vi "error handler - SubVI.vi"(4 "error in":errorcluster, 7 "Dialog box?":bool=TRUE) -> (0 "error out":errorcluster, 2 "message":string=" INSTRUCTIONS:\r\rNormal Use:  When using subVIs that incorporate the error in/error out (or error I/O) structure, place this handler where you want to inform the user of an error, typically at the end of the I/O data path, as the last action of the program.  If the error in error? is ERROR, the handler creates a message describing the error and its source.  If the type of dialog = 1 (default), the message is displayed to the user, who can only acknowedge it.  If the type = 2, the user can acknowledge the message or abort execution; aborting a program with active I/O is not recommended.  If the type = 0, no message is displayed; this is used to process the error programmatically, and the error out cluster elements are wired to individual terminals for that reason.  \r\rOther Use:\n\r\nlocal testing.  To test the error code of a subVI or function that does not have the error I/O structure, you can wire its error code and a source string to the local error code and error source inputs.  If error in error? indicates no error and error code is not equal to 0, the local code and source are substituted for the error in values, and error? is set TRUE (ERROR).", 3 "no error out":errorcluster)   [LabVIEW 2014]
uses:
  Lambda Globals.vi
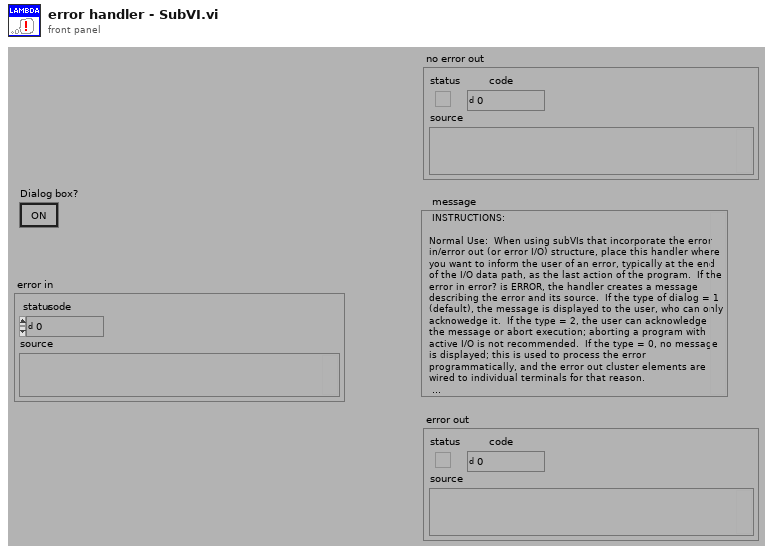
[diagram p1: front panel]
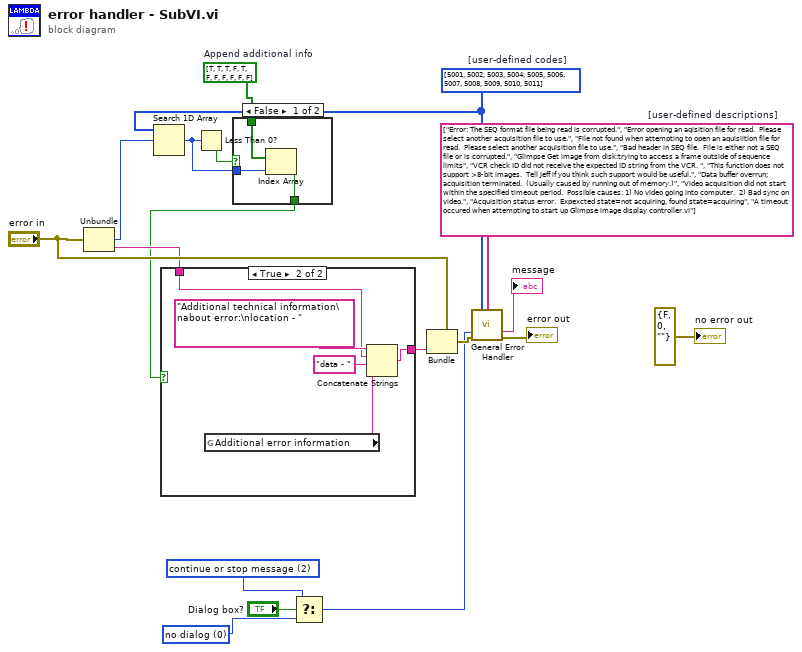
[diagram p0: block diagram]
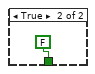
[diagram p2: hidden frame]
diagram:
  w5 = u16 2 items=["no dialog", "OK message", "continue or stop message"] ("type of dialog (OK msg:1)")
  w4 = u16 0 items=["no dialog", "OK message", "continue or stop message"] ("type of dialog (OK msg:1)")
  w8 = bool[] [TRUE, TRUE, TRUE, FALSE, TRUE, FALSE, FALSE, FALSE, FALSE, FALSE, FALSE]  # Append additional info
  w17 = string[] ["Error: The SEQ format file being read is corrupted.", "Error opening an aqisition file for read.  Please select another acquisition file to use.", "File not found when attempting to open an aquisiition file for read.  Please select another acquisition file to use.", "Bad header in SEQ file.  File is either not a SEQ file or is corrupted.", "Glimpse Get image from disk:trying to access a frame outside of sequence limits", "VCR check ID did not receive the expected ID string from the VCR. ", "This function does not support >8-bit images.  Tell Jeff if you think such support would be useful.", "Data buffer overrun; acquisition terminated.  (Usually caused by running out of memory.)", "Video acquisition did not start within the specified timeout period.  Possible causes: 1) No video going into computer.  2) Bad sync on video.", "Acquisition status error.  Expexcted state=not acquiring, found state=acquiring", "A timeout occured when attempting to start up Glimpse image display controller.vi"]  # [user-defined descriptions]
  w11 = i32[] [5001, 5002, 5003, 5004, 5005, 5006, 5007, 5008, 5009, 5010, 5011]  # [user-defined codes]
  n1 = Unbundle("error in") -> ("code"=w10:i32, "source"=w13:string)  [unwired: 1 out]
  n2 = Search 1D Array(1D array=w11, element=w10) -> (index of element=w7:i32)  [unwired: 1 out]
  n3 = Less Than 0?(x=w7) -> (x < 0?=w9:bool)
  n4 = case shown="False" w9 {
    tunnel: w8 -> [w21 _]
    tunnel: w7 -> [w20 _]
    tunnel: [w19 FALSE] -> w6
    frame False {
      n5 = Index Array(array=w21, index=w20) -> (element=w19:bool)
    }
    frame True {
    }
  }
  n6 = case shown="True" w6 {
    tunnel: w13 -> [w23 w26]
    tunnel: [w23 w28] -> w12
    frame False {
    }
    frame True {
      n7 = global read "Lambda Globals.vi" "Additional error information"() -> (w24:string)
      n8 = Concatenate Strings("Additional technical information\nabout error:\nlocation - " ("string"), w26, "data - " ("string"), w24) -> (w28:string)
    }
  }
  n9 = Select(t=w5, s="Dialog box?", f=w4) -> (s? t:f=w2:u16)
  n10 = Bundle(cluster="error in", "source"=w12) -> (w15:errorcluster)  [unwired: 2 out]
  n11 = call <vilib>:"General Error Handler.vi"("[user-defined codes]"=w11, "[user-defined descriptions]"=w17, "type of dialog (OK msg:1)"=w2, "error in (no error)"=w15) -> ("message"=→"message":string, "error out"=→"error out":errorcluster)  [unwired: 1 in, 9 out]
  "no error out" <- errorcluster {"status"=FALSE, "code"=0, "source"=""} ("no error out")
